vi "INIT.vi"(8 "error in (no error)":errorcluster, 11 "Control-Client in":refnum<class "Control-Client.lvclass">) -> (0 "error out":errorcluster, 3 "Control-Client out":refnum<class "Control-Client.lvclass">)   [LabVIEW 2019, in "Control-Client.lvclass"]
uses:
  Control-Client.lvclass
  C:/dev/TRANCON/Classes/GeneralFunctionality/GeneralFunctionality.lvclass
  Config/Config.lvclass
  Config/config_names_def.ctl
  GeneralFunctionality/GeneralFunctionality.lvclass/GeneralFunctionality.ctl
  Control-Client.lvclass/Control-Client.ctl
  dependecies/ControlsVIs/Clusters-def/Message types.ctl
  Message/Message.lvclass
  Message/Message.lvclass/Message.ctl
  GeneralFunctionality/GeneralFunctionality.lvclass
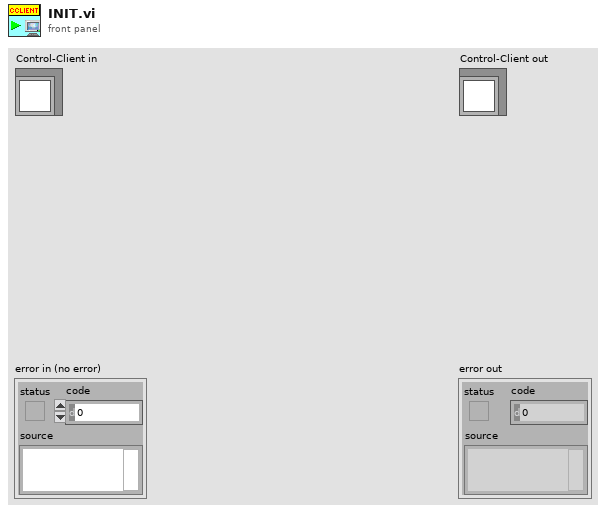
[diagram p1: front panel]
types:
  T1 = typedef "Config.lvclass/config_names_def.ctl" = string
  T2 = typedef "Message types.ctl" = string
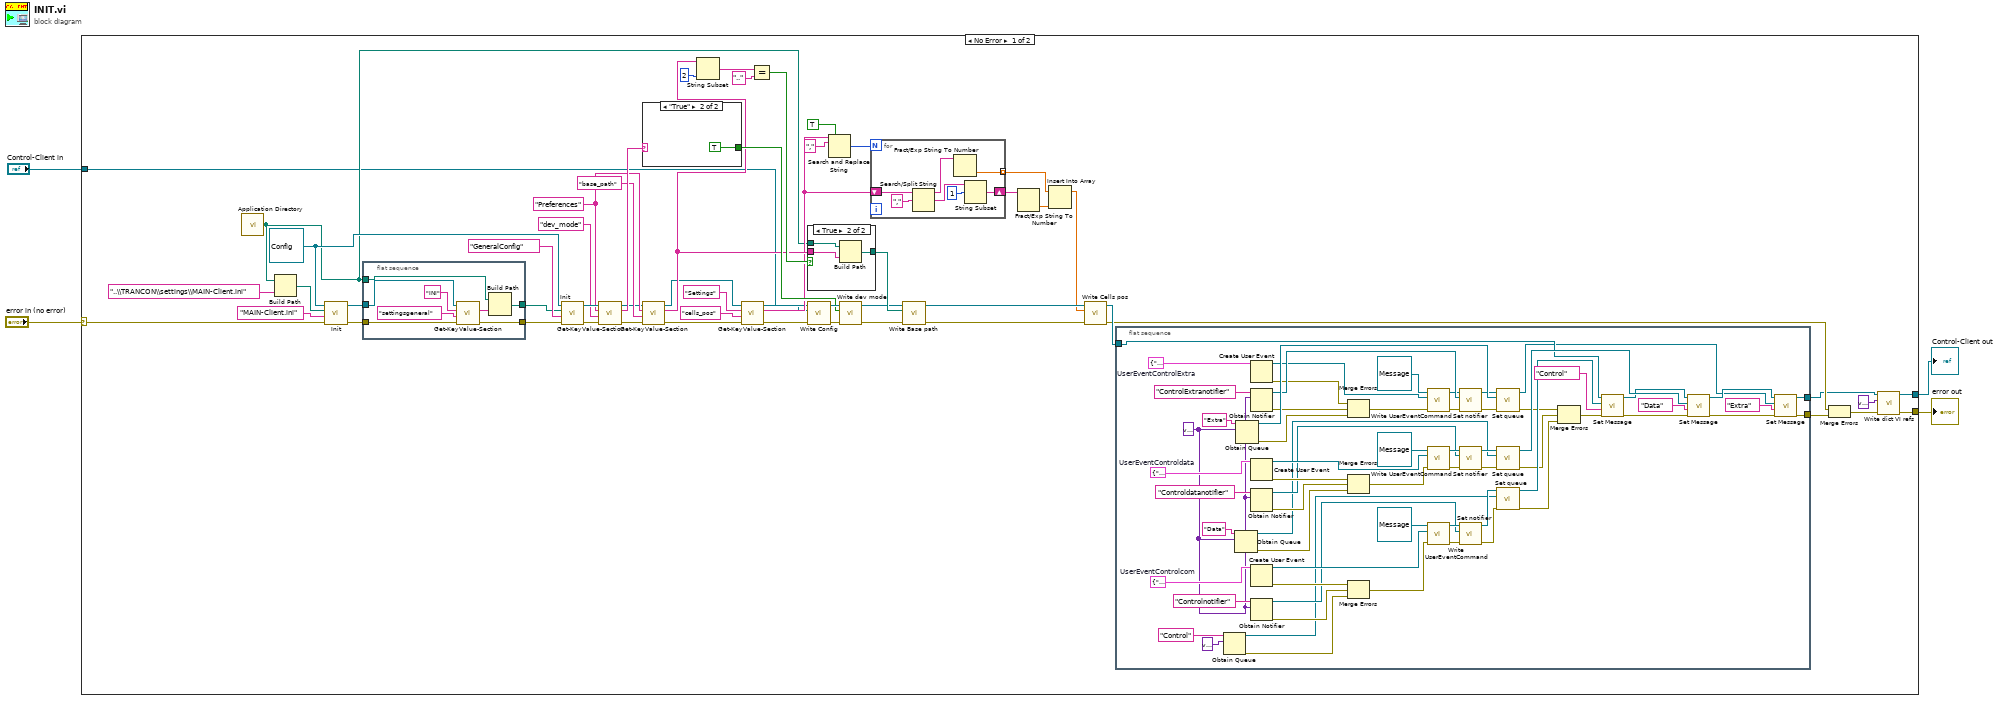
[diagram p0: block diagram]
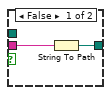
[diagram p2: hidden frame]
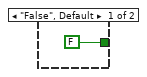
[diagram p3: hidden frame]
diagram:
  n1 = case shown="No Error" "error in (no error)" {
    selector: "error in (no error)" -> [w32 w147]
    tunnel: [w11 w147] -> w2
    tunnel: "Control-Client in" -> [w13 w146]
    tunnel: [w9 w146] -> w1
    frame No Error {
      w42 = "Preferences" ("Section")
      w53 = refnum<class "Config.lvclass"> refnum ("Config.lvclass")
      n2 = call <vilib>:"Application Directory.vi"() -> ("Application Directory"=w14:path)
      n3 = Build Path(base path=w14, name or relative path="..\\TRANCON\\settings\\MAIN-Client.ini" ("nom ou chemin relatif")) -> (appended path=w57:path)
      n4 = call "Init.vi"("error in"=w32, "Name"="MAIN-Client.ini", "Path"=w57, "Config in"=w53) -> ("error out"=w55:errorcluster, "Config out"=w56:refnum<class "Config.lvclass">)  [unwired: 6 in]
      n5 = flat-sequence {
        tunnel: w56 -> [w145]
        tunnel: w55 -> [w144]
        tunnel: w14 -> [w140]
        tunnel: [w139] -> w51
        tunnel: [w138] -> w52
        frame #0 {
          n6 = call-dynamic "Get-KeyValue-Section.vi"("error in (no error)"=w144, "Key"="settingsgeneral", "Section"="INI", "Config in"=w145) -> ("error out"=w139:errorcluster, "Value"=w141:string)  [unwired: 5 in, 1 out]
          n7 = Build Path(base path=w140, name or relative path=w141) -> (appended path=w138:path)
        }
      }
      n8 = call "Init.vi"("error in"=w51, "Name"=T1 "GeneralConfig" ("Combo Box"), "Path"=w52, "Config in"=w53) -> ("error out"=w48:errorcluster, "Config out"=w50:refnum<class "Config.lvclass">)  [unwired: 6 in]
      n9 = call-dynamic "Get-KeyValue-Section.vi"("error in (no error)"=w48, "Key"="dev_mode", "Section"=w42, "Config in"=w50) -> ("error out"=w40:errorcluster, "Value"=w47:string, "Config out"=w39:refnum<class "Config.lvclass">)  [unwired: 5 in]
      n10 = case shown="\"True\"" w47 {
        tunnel: [FALSE TRUE] -> w44
        frame "False", Default {
        }
        frame "True" {
        }
      }
      n11 = call-dynamic "Get-KeyValue-Section.vi"("error in (no error)"=w40, "Key"="base_path", "Section"=w42, "Config in"=w39) -> ("error out"=w23:errorcluster, "Value"=w34:string, "Config out"=w26:refnum<class "Config.lvclass">)  [unwired: 5 in]
      n12 = String Subset(string=w34, length (rest)=2 ("length (rest)")) -> (substring=w37:string)  [unwired: 1 in]
      n13 = call-dynamic "Get-KeyValue-Section.vi"("error in (no error)"=w23, "Key"="cells_pos", "Section"="Settings", "Config in"=w26) -> ("error out"=w5:errorcluster, "Value"=w16:string, "Config out"=w6:refnum<class "Config.lvclass">)  [unwired: 5 in]
      n14 = Equal?(x=w37, y=".." ("x")) -> (x = y?=w35:bool)
      n15 = case shown="True" w35 {
        tunnel: w14 -> [_ w71]
        tunnel: w34 -> [w68 w70]
        tunnel: [w67 w69] -> w33
        frame False {
          n16 = String To Path(string=w68) -> (path=w67:path)
        }
        frame True {
          n17 = Build Path(base path=w71, name or relative path=w70) -> (appended path=w69:path)
        }
      }
      n18 = call "Write Config.vi"("error in (no error)"=w5, "Config.lvclass"=w6, "GeneralFunctionality en entrée"=w13) -> ("error out"=w46:errorcluster, "GeneralFunctionality en sortie"=w45:refnum<class "Control-Client.lvclass">)  [unwired: 7 in]
      n19 = Search and Replace String(replace all?=TRUE ("replace all? (F)"), input string=w16, search string=",") -> (number of replacements=w21:i32)  [unwired: 5 in, 3 out]
      n20 = call "Write dev mode.vi"("error in (no error)"=w46, "Dev_mode"=w44, "Control-Client in"=w45) -> ("error out"=w30:errorcluster, "Control-Client out"=w31:refnum<class "Control-Client.lvclass">)  [unwired: 7 in]
      n21 = for {
        N: w21 -> [_]
        tunnel: [w60] -> w19 mode=indexing
        shift-right: [w62] -> w18
        shift-left: w16 -> [w65]
        n22 = Search/Split String(string=w65, search string/char (-)=",") -> (substring before match=w61:string, match + rest of string=w64:string)  [unwired: 1 in, 1 out]
        n23 = Fract/Exp String To Number(string=w61) -> (number=w60:dbl)  [unwired: 3 in, 1 out]
        n24 = String Subset(string=w64, offset (0)=1) -> (substring=w62:string)  [unwired: 1 in]
      }
      n25 = call "Write Base path.vi"("error in (no error)"=w30, "Base path"=w33, "Control-Client in"=w31) -> ("error out"=w29:errorcluster, "Control-Client out"=w28:refnum<class "Control-Client.lvclass">)  [unwired: 7 in]
      n26 = Fract/Exp String To Number(string=w18) -> (number=w17:dbl)  [unwired: 3 in, 1 out]
      n27 = Insert Into Array(array=w19, new element=w17) -> (w15:dbl[])  [unwired: 1 in]
      n28 = call "Write Cells pos.vi"("error in (no error)"=w29, "Cells pos"=w15, "Control-Client in"=w28) -> ("error out"=w10:errorcluster, "Control-Client out"=w27:refnum<class "Control-Client.lvclass">)  [unwired: 7 in]
      n29 = flat-sequence {
        tunnel: w27 -> [w100]
        tunnel: [w80] -> w8
        tunnel: [w81] -> w43
        frame #0 {
          w88 = cluster{"command":string, "data":variant} {"command"="", "data"=variant}  # UserEventControlExtra
          w116 = cluster{"command":string, "data":variant} {"command"="", "data"=variant}  # UserEventControldata
          w76 = variant
          w131 = cluster{"command":string, "data":variant} {"command"="", "data"=variant}  # UserEventControlcom
          n30 = Obtain Queue(name (unnamed)="Control", element data type=variant) -> (queue out=w106:refnum<queue>, error out=w112:errorcluster)  [unwired: 3 in, 1 out]
          n31 = Obtain Queue(name (unnamed)="Data", element data type=w76) -> (queue out=w105:refnum<queue>, error out=w111:errorcluster)  [unwired: 3 in, 1 out]
          n32 = Obtain Queue(name (unnamed)="Extra", element data type=w76) -> (queue out=w94:refnum<queue>, error out=w73:errorcluster)  [unwired: 3 in, 1 out]
          n33 = Create User Event(user event datatype=w88) -> (user event=w91:refnum<user-event>, error out=w90:errorcluster)  [unwired: 1 in]
          n34 = Obtain Notifier(name (unnamed)="ControlExtranotifier" ("nom (aucun)"), notification data type=w76) -> (notifier out=w92:refnum<notifier>, error out=w74:errorcluster)  [unwired: 2 in, 1 out]
          n35 = Create User Event(user event datatype=w116) -> (user event=w109:refnum<user-event>, error out=w114:errorcluster)  [unwired: 1 in]
          n36 = Obtain Notifier(name (unnamed)="Controldatanotifier" ("nom (aucun)"), notification data type=w76) -> (notifier out=w108:refnum<notifier>, error out=w113:errorcluster)  [unwired: 2 in, 1 out]
          n37 = Create User Event(user event datatype=w131) -> (user event=w133:refnum<user-event>, error out=w129:errorcluster)  [unwired: 1 in]
          n38 = Obtain Notifier(name (unnamed)="Controlnotifier" ("nom (aucun)"), notification data type=w76) -> (notifier out=w127:refnum<notifier>, error out=w128:errorcluster)  [unwired: 2 in, 1 out]
          n39 = Merge Errors(w90, w74, w73) -> (w72:errorcluster)
          n40 = Merge Errors(w114, w113, w111) -> (w110:errorcluster)
          n41 = Merge Errors(w129, w128, w112) -> (w126:errorcluster)
          n42 = call "Write UserEventCommand.vi"("error in (no error)"=w72, "UserEventCommand"=w91, "Message en entrée"=refnum<class "Message.lvclass"> refnum ("Message.lvclass")) -> ("error out"=w84:errorcluster, "Message en sortie"=w85:refnum<class "Message.lvclass">)  [unwired: 7 in]
          n43 = call "Write UserEventCommand.vi"("error in (no error)"=w110, "UserEventCommand"=w109, "Message en entrée"=refnum<class "Message.lvclass"> refnum ("Message.lvclass")) -> ("error out"=w120:errorcluster, "Message en sortie"=w119:refnum<class "Message.lvclass">)  [unwired: 7 in]
          n44 = call "Write UserEventCommand.vi"("error in (no error)"=w126, "UserEventCommand"=w133, "Message en entrée"=refnum<class "Message.lvclass"> refnum ("Message.lvclass")) -> ("error out"=w130:errorcluster, "Message en sortie"=w134:refnum<class "Message.lvclass">)  [unwired: 7 in]
          n45 = call "Set notifier.vi"("error in (no error)"=w84, "notifier"=w92, "Message en entrée"=w85) -> ("error out"=w93:errorcluster, "Message en sortie"=w87:refnum<class "Message.lvclass">)  [unwired: 7 in]
          n46 = call "Set notifier.vi"("error in (no error)"=w120, "notifier"=w108, "Message en entrée"=w119) -> ("error out"=w107:errorcluster, "Message en sortie"=w117:refnum<class "Message.lvclass">)  [unwired: 7 in]
          n47 = call "Set notifier.vi"("error in (no error)"=w130, "notifier"=w127, "Message en entrée"=w134) -> ("error out"=w123:errorcluster, "Message en sortie"=w124:refnum<class "Message.lvclass">)  [unwired: 7 in]
          n48 = call "Set queue.vi"("error in (no error)"=w93, "queue"=w94, "Message in"=w87) -> ("error out"=w77:errorcluster, "Message out"=w78:refnum<class "Message.lvclass">)  [unwired: 7 in]
          n49 = call "Set queue.vi"("error in (no error)"=w107, "queue"=w105, "Message in"=w117) -> ("error out"=w98:errorcluster, "Message out"=w102:refnum<class "Message.lvclass">)  [unwired: 7 in]
          n50 = call "Set queue.vi"("error in (no error)"=w123, "queue"=w106, "Message in"=w124) -> ("error out"=w97:errorcluster, "Message out"=w103:refnum<class "Message.lvclass">)  [unwired: 7 in]
          n51 = Merge Errors(w77, w98, w97) -> (w96:errorcluster)
          n52 = call "Set Message.vi"("error in (no error)"=w96, "Message type"=T2 "Control", "Message.lvclass"=w103, "GeneralFunctionality en entrée"=w100) -> ("error out"=w95:errorcluster, "GeneralFunctionality en sortie"=w101:refnum<class "Control-Client.lvclass">)  [unwired: 6 in]
          n53 = call "Set Message.vi"("error in (no error)"=w95, "Message type"=T2 "Data", "Message.lvclass"=w102, "GeneralFunctionality en entrée"=w101) -> ("error out"=w82:errorcluster, "GeneralFunctionality en sortie"=w79:refnum<class "Control-Client.lvclass">)  [unwired: 6 in]
          n54 = call "Set Message.vi"("error in (no error)"=w82, "Message type"=T2 "Extra", "Message.lvclass"=w78, "GeneralFunctionality en entrée"=w79) -> ("error out"=w81:errorcluster, "GeneralFunctionality en sortie"=w80:refnum<class "Control-Client.lvclass">)  [unwired: 6 in]
        }
      }
      n55 = Merge Errors(w10, w43) -> (w12:errorcluster)
      n56 = call "Write dict VI refs.vi"("error in (no error)"=w12, "VI refs"=variant, "Control-Client in"=w8) -> ("error out"=w11:errorcluster, "Control-Client out"=w9:refnum<class "Control-Client.lvclass">)  [unwired: 7 in]
    }
    frame Error {
    }
  }
  "error out" <- w2
  "Control-Client out" <- w1
